vi "testvideo.vi"() -> ()   [LabVIEW 2012]
uses:
  <vilib>/userdefined/High Color/IMAQdx.ctl
  <vilib>/vision/driver/NI_Vision_Acquisition_Software.lvlib
panel:
  out "image":T1(plugin-control)
  in  "stop":bool
  in  "Session In":T2
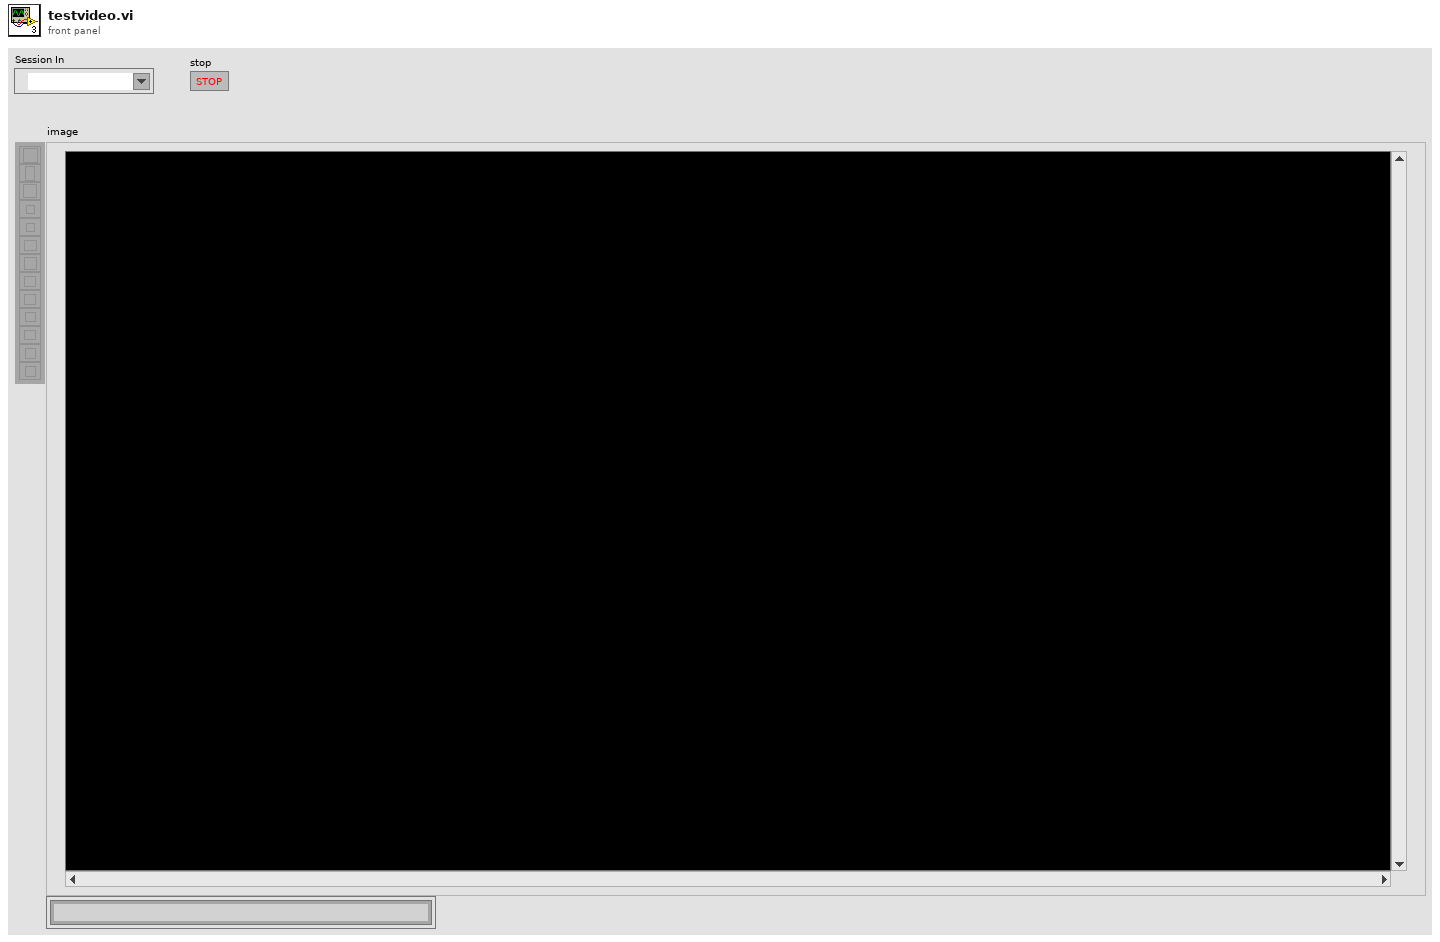
[diagram p1: front panel]
types:
  T1 = typedef "IMAQ Image.ctl" = refnum<image>
  T2 = typedef "IMAQdx.ctl" = refnum<k21>
  T3 = typedef "Image Type" = u32
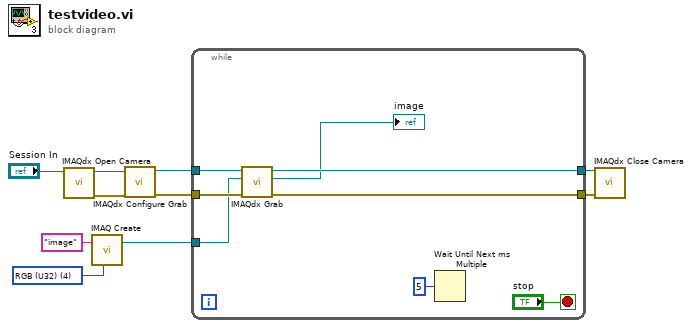
[diagram p0: block diagram]
diagram:
  w1 = T3 4 items=["Grayscale (U8)", "Grayscale (I16)", "Grayscale (SGL)", "Complex (CSG)", "RGB (U32)", "HSL (U32)", "RGB (U64)", "Grayscale (U16)"] ("Image Type")
  n1 = call <vilib>:"IMAQdx Open Camera.vi"("Session In"="Session In") -> ("error out"=w8:errorcluster, "Session Out"=w9:T2)  [unwired: 9 in]
  n2 = call "IMAQ Create"("Image Name"="image", "Image Type"=w1) -> ("New Image"=w2:T1)  [unwired: 3 in, 1 out]
  n3 = call <vilib>:"IMAQdx Configure Grab.vi"("error in"=w8, "Session In"=w9) -> ("error out"=w6:errorcluster, "Session Out"=w7:T2)  [unwired: 8 in]
  n4 = while {
    tunnel: w7 -> [w18]
    tunnel: w6 -> [w17]
    tunnel: [w15] -> w5
    tunnel: [w14] -> w4
    tunnel: w2 -> [w12]
    stop <- "stop" stop-if-true
    n5 = call <vilib>:"IMAQdx Grab.vi"("error in"=w17, "Image In"=w12, "Session In"=w18) -> ("error out"=w14:errorcluster, "Image Out"=→"image":T1, "Session Out"=w15:T2)  [unwired: 5 in, 1 out]
    n6 = Wait Until Next ms Multiple(millisecond multiple=u32 5) -> ()  [unwired: 1 out]
  }
  n7 = call <vilib>:"IMAQdx Close Camera.vi"("error in"=w4, "Session In"=w5) -> ()  [unwired: 9 in, 1 out]
